vi "Test.Maui 2.0.Initialize.Plenty.Subpanels.Subpanel 2.vi"(8 "error in":errorcluster) -> (0 "error out":errorcluster)   [LabVIEW 2019]
uses:
  Maui 2.0/Maui 2.0.lvclass
  <vilib>/JKI/JKI SMO/SMO/SMO.lvclass
  Helper/Test Helper 1/Test Helper 1.lvclass
  <vilib>/addons/_JKI Toolkits/Caraya/classes/Test/Test.lvclass
  <vilib>/addons/_JKI Toolkits/Caraya/classes/Assert/Assert.lvclass
  C:/Program Files (x86)/National Instruments/LabVIEW 2019/vi.lib/JKI/JKI SMO/SMO/SMO.lvclass
  <vilib>/addons/_JKI Toolkits/Caraya/classes/Assert/Assert Equal Value_Variant.vi
panel:
  in  "Ring 2":u16(ring) items=["Test Helper 1", "Test Helper 1", "Maui 2.0", "None"]
  in  "Ring":u16(ring) items=["Test Helper 1", "Test Helper 1", "Maui 2.0", "None"]
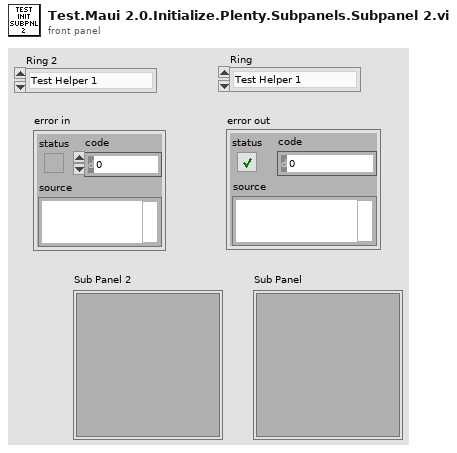
[diagram p1: front panel]
types:
  T1 = cluster{"Ring":refnum<vi>, "Sub Panel":refnum<vi>}
  T2 = cluster{"Ring 2":refnum<vi>, "Sub Panel 2":refnum<vi>}
  T3 = cluster{"Ring 2":refnum<vi>, "Sub Panel 2":refnum<vi>}[]
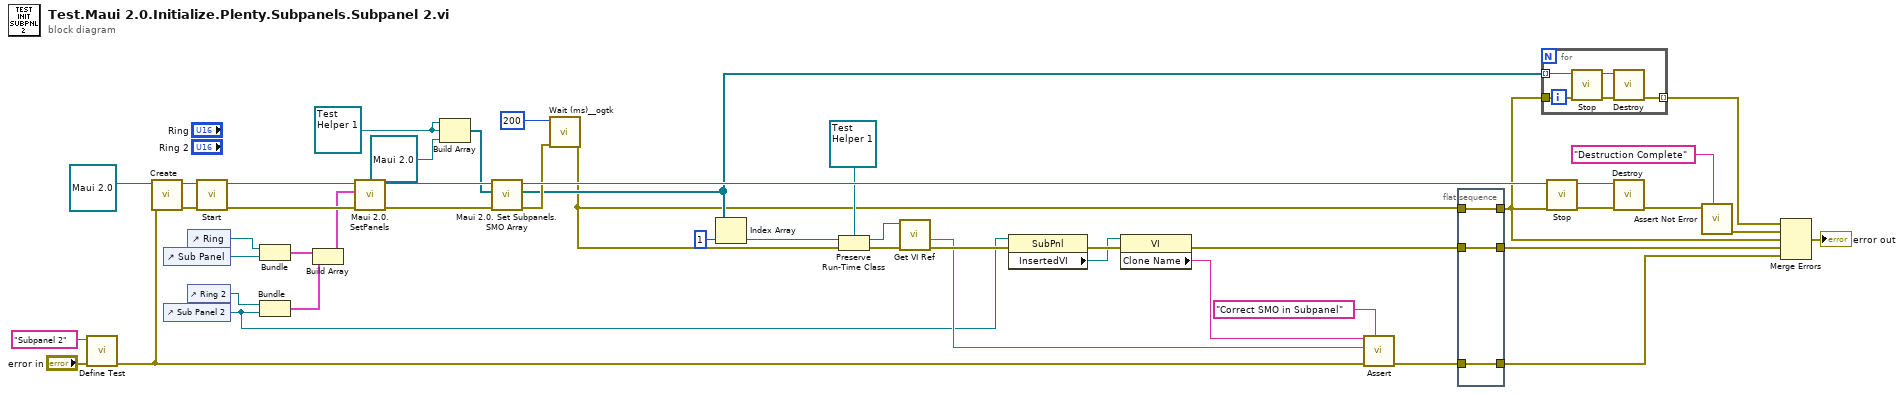
[diagram p0: block diagram]
diagram:
  w18 = refnum<class "Test Helper 1.lvclass"> refnum ("Test Helper 1.lvclass")
  n1 = call <vilib>:"Define Test.vi"("error in (no error)"="error in", "Label (VI Title)"="Subpanel 2") -> ("error out"=w21:errorcluster)  [unwired: 9 in]
  n2 = call <vilib>:"Create.vi"("error in (no error)"=w21, "SMO"=refnum<class "Maui 2.0.lvclass"> refnum ("Maui 2.0 in")) -> ("error out"=w48:errorcluster, "SMO out"=w42:refnum<class "Maui 2.0.lvclass">)  [unwired: 7 in, 1 out]
  n3 = control-ref of="Sub Panel"() -> (w10:refnum<vi>)
  n4 = control-ref of="Sub Panel 2"() -> (w1:refnum<vi>)
  n5 = control-ref of="Ring"() -> (w35:refnum<vi>)
  n6 = control-ref of="Ring 2"() -> (w45:refnum<vi>)
  n7 = call <vilib>:"Start.vi"("error in (no error)"=w48, "SMO"=w42) -> ("error out"=w47:errorcluster, "SMO out"=w40:refnum<class "Maui 2.0.lvclass">)  [unwired: 8 in]
  n8 = Bundle("Ring"=w35, "Sub Panel"=w10) -> (w44:T1)  [unwired: 1 in]
  n9 = Bundle("Ring 2"=w45, "Sub Panel 2"=w1) -> (w43:T2)  [unwired: 1 in]
  n10 = Build Array(w44, w43) -> (w36:T3)
  n11 = call "Maui 2.0.SetPanels.vi"("error in (no error)"=w47, "Set Panels"=w36, "Maui 2.0"=w40) -> ("error out"=w46:errorcluster, "Maui 2.0 out"=w39:refnum<class "Maui 2.0.lvclass">)  [unwired: 7 in]
  n12 = Build Array(w18, w18, refnum<class "Maui 2.0.lvclass"> refnum ("Maui 2.0 in")) -> (w37:refnum<class "SMO.lvclass">[])
  n13 = call-dynamic "Maui 2.0. Set Subpanels.SMO Array.vi"("error in (no error)"=w46, "Subpanels in"=w37, "Maui 2.0 in"=w39) -> ("error out"=w24:errorcluster, "Subpanels Out"=w6:refnum<class "SMO.lvclass">[], "Maui 2.0 out"=w32:refnum<class "Maui 2.0.lvclass">)  [unwired: 6 in]
  n14 = call <userlib>:"Wait (ms)__ogtk.vi"("error in (no error)"=w24, "milliseconds to wait"=u32 200) -> ("error out"=w5:errorcluster)  [unwired: 8 in, 1 out]
  n15 = Index Array(array=w6, index=1) -> (element=w20:refnum<class "SMO.lvclass">)
  n16 = Preserve Run-Time Class(object in=w20, error in=w5, 2:refnum<class "Test Helper 1.lvclass"> refnum ("Test Helper 1.lvclass")) -> (object out=w17:refnum<class "Test Helper 1.lvclass">, error out=w16:errorcluster)
  n17 = call-dynamic "Get VI Ref.vi"("error in (no error)"=w16, "Test Helper 1 in"=w17) -> ("error out"=w15:errorcluster, "VI Clone Name"=w4:string)  [unwired: 6 in, 2 out]
  n18 = property on="Property Node" class="SubPnl"(reference=w1, error in=w15) -> (error out=w13:errorcluster, "InsertedVI"=w11:refnum<vi>)  [unwired: 1 out]
  n19 = property on="Property Node" class="VI"(reference=w11, error in=w13) -> (error out=w12:errorcluster, "Clone Name"=w8:string)  [unwired: 1 out]
  n20 = call-poly <vilib>:"Assert.vi"("Label"="Correct SMO in Subpanel", "error in (no error)"=w21, "Y"=w4, "X"=w8) -> ("error out"=w9:errorcluster)  [unwired: 7 in]
  n21 = flat-sequence {
    tunnel: w5 -> [w51]
    tunnel: w12 -> [w50]
    tunnel: w9 -> [w49]
    tunnel: [w51] -> w22
    tunnel: [w50] -> w26
    tunnel: [w49] -> w25
    frame #0 {
    }
  }
  n22 = for {
    tunnel: w6 -> [w55] mode=indexing
    tunnel: w22 -> [w54]
    tunnel: [w52] -> w23 mode=indexing
    n23 = call <vilib>:"Stop.vi"("error in (no error)"=w54, "SMO"=w55) -> ("error out"=w53:errorcluster, "SMO out"=w56:refnum<class "SMO.lvclass">)  [unwired: 8 in]
    n24 = call <vilib>:"Destroy.vi"("error in (no error)"=w53, "SMO"=w56) -> ("error out"=w52:errorcluster)  [unwired: 9 in]
  }
  n25 = call <vilib>:"Stop.vi"("error in (no error)"=w22, "SMO"=w32) -> ("error out"=w30:errorcluster, "SMO out"=w31:refnum<class "Maui 2.0.lvclass">)  [unwired: 8 in]
  n26 = call <vilib>:"Destroy.vi"("error in (no error)"=w30, "SMO"=w31) -> ("error out"=w29:errorcluster)  [unwired: 9 in]
  n27 = call <vilib>:"Assert Not Error.vi"("Label"="Destruction Complete", "Not Error?"=w29) -> ("error out"=w27:errorcluster)  [unwired: 9 in]
  n28 = Merge Errors(w23, w27, w22, w26, w25) -> (→"error out":errorcluster)
